vi "ultima aula pisca pisca 12 02 kk.vi"() -> ()   [LabVIEW 2024]
uses:
  <vilib>/Instr/_visa.llb/VISA Configure Serial Port (Instr).vi
panel:
  in  "write buffer":string
  in  "Numeric 2":i32
  out "Humidade":dbl(graph)
  out "output 2":dbl
  out "read buffer 3":string
  out "output 1":dbl
  out "Temperatura":dbl(graph)
  in  "termination char\n(0xA = '\\n' = LF)":u8=10 format="%.0x"
  in  "VISA resource name":refnum<visa-resource-name>
  in  "stop":bool
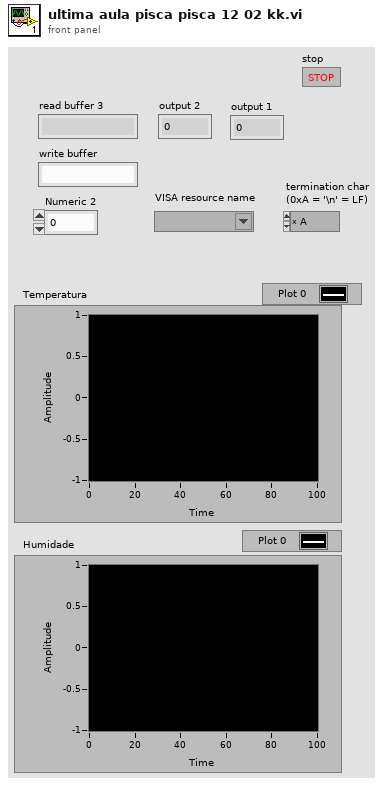
[diagram p1: front panel]
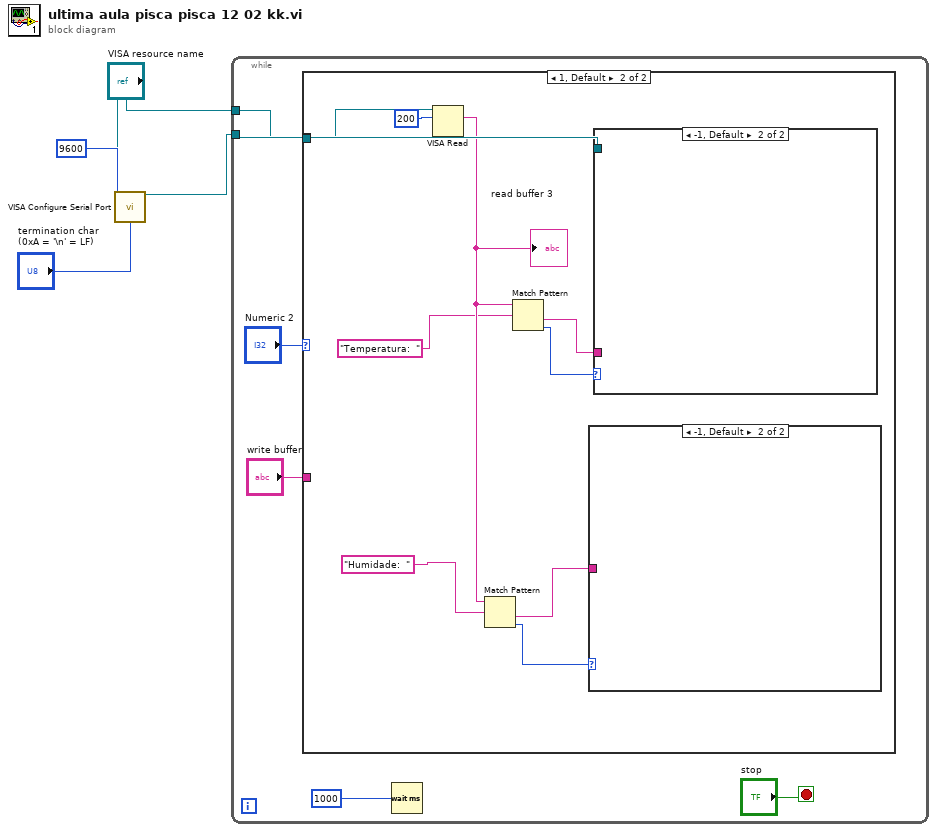
[diagram p0: block diagram]
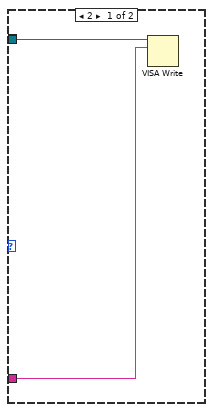
[diagram p2: hidden frame]
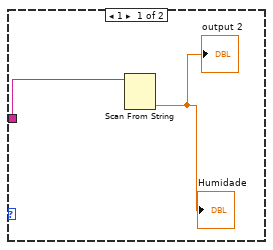
[diagram p3: hidden frame]
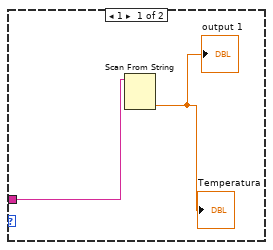
[diagram p4: hidden frame]
diagram:
  n1 = call-poly "VISA Configure Serial Port"("VISA resource name"="VISA resource name", "termination char\n(0xA = '\\n' = LF)"="termination char\n(0xA = '\\n' = LF)", "baud rate (9600)"=u32 9600) -> ("VISA resource name out"=w3:refnum<visa-resource-name>)  [unwired: 11 in, 1 out]
  n2 = while {
    tunnel: w3 -> [w9]
    tunnel: "VISA resource name" -> [w7]
    stop <- "stop" stop-if-true
    n3 = case shown="1, Default" "Numeric 2" {
      tunnel: w9 -> [w12 w22]
      tunnel: w7 -> [_ w20]
      tunnel: "write buffer" -> [w11 _]
      frame 2 {
        n4 = VISA Write(VISA resource name=w12, write buffer=w11) -> ()  [unwired: 1 in, 3 out]
      }
      frame 1, Default {
        n5 = VISA Read(VISA resource name=w20, byte count=u32 200) -> (read buffer=w17:string)  [unwired: 1 in, 3 out]
        "read buffer 3" <- w17
        n6 = Match Pattern(string=w17, regular expression="Humidade:  ") -> (after substring=w15:string, offset past match=w14:i32)  [unwired: 1 in, 2 out]
        n7 = Match Pattern(string=w17, regular expression="Temperatura:  ") -> (after substring=w18:string, offset past match=w19:i32)  [unwired: 1 in, 2 out]
        n8 = case shown="-1, Default" w14 {
          tunnel: w15 -> [w23 _]
          frame 1 {
            n9 = Scan From String(input string=w23) -> (output 1=→"Humidade" →"output 2":dbl)  [unwired: 4 in, 3 out]
          }
          frame -1, Default {
          }
        }
        n10 = case shown="-1, Default" w19 {
          tunnel: w22 -> [_ _]
          tunnel: w18 -> [w25 _]
          frame 1 {
            n11 = Scan From String(input string=w25) -> (output 1=→"Temperatura" →"output 1":dbl)  [unwired: 4 in, 3 out]
          }
          frame -1, Default {
          }
        }
      }
    }
    n12 = Wait (ms)(milliseconds to wait=u32 1000) -> ()  [unwired: 1 out]
  }
